vi "set pixel line.vi"(7 "dy":dbl, 8 "error in (no error)":errorcluster, 9 "dx":dbl, 10 "pixelperiod":u16, 11 "pixelmode":u16) -> (0 "error out":errorcluster)   [LabVIEW 2015, in "SCANalone4x64.lvlib"]
doc: "__declspec(dllimport) void __stdcall set_pixel_line(unsigned short pixelmode, unsigned short pixelperiod, double dx, double dy);"
uses:
  <userlib>/SCANalone4x64/SCANalone4x64.lvlib
  <userlib>/SCANalone4x64/SCANalone4x64.dll
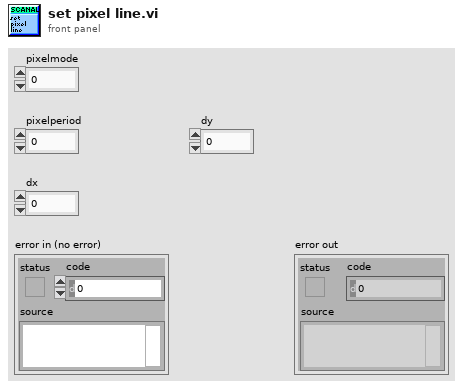
[diagram p1: front panel]
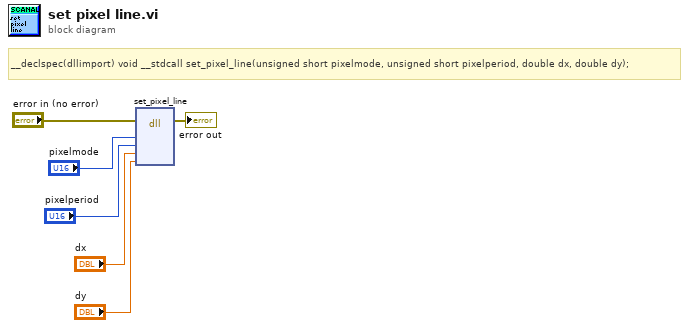
[diagram p0: block diagram]
diagram:
  # "__declspec(dllimport) void __stdcall set_pixel_line(unsigned short pixelmode, unsigned short pixelperiod, double dx, double dy);"
  n1 = dll-call lib="C:/Program Files/National Instruments/LabVIEW 2015/user.lib/SCANalone4x64/SCANalone4x64.*" fn="set_pixel_line"(error in="error in (no error)", "pixelmode"="pixelmode", "pixelperiod"="pixelperiod", "dx"="dx", "dy"="dy") -> (error out=→"error out":errorcluster)  [unwired: 7 in, 1 out]
